vi "Parse IDN String.vi"(5 "error in (no error)":errorcluster, 6 "IDN String":string) -> (0 "error out":errorcluster, 1 "Info":string, 2 "Model":string, 3 "Manufacturer":string, 4 "Revision":string)   [LabVIEW 2019]
uses:
  New NML Data Acq/SubVIs/NML Data Acq Globals.vi
  <vilib>/regexp/Match Regular Expression.xnode
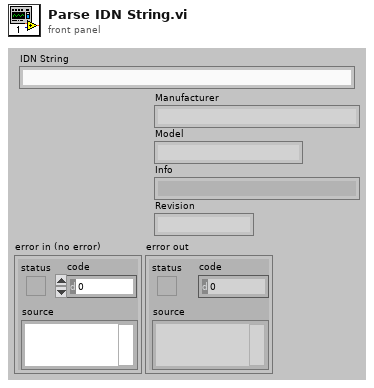
[diagram p1: front panel]
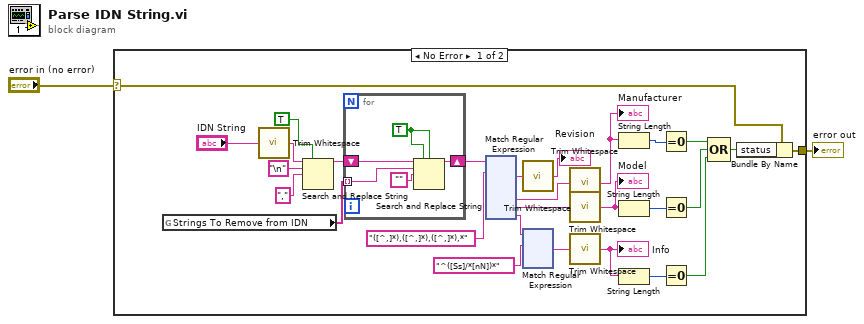
[diagram p0: block diagram]
diagram:
  n1 = case shown="No Error" "error in (no error)" {
    selector: "error in (no error)" -> [w24 w262]
    tunnel: [w23 w262] -> w1
    frame No Error {
      n2 = global read "NML Data Acq Globals.vi" "Strings To Remove from IDN"() -> (w22:string[])
      n3 = call <vilib>:"Trim Whitespace.vi"("string"="IDN String") -> ("trimmed string"=w3:string)  [unwired: 1 in]
      n4 = Search and Replace String(replace all?=TRUE ("replace all? (F)"), input string=w3, search string="\n", replace string="," ("replace string (\"\")")) -> (result string=w26:string)  [unwired: 4 in, 3 out]
      n5 = for {
        tunnel: w22 -> [w259] mode=indexing
        shift-right: [w260] -> w9
        shift-left: w26 -> [w261]
        w258 = TRUE ("replace all? (F)")
        n6 = Search and Replace String(replace all?=w258, case sensitive?=w258, input string=w261, search string=w259, replace string="") -> (result string=w260:string)  [unwired: 3 in, 3 out]
      }
      n7 = xnode "Match Regular Expression"("input string"=w9, "regular expression"="([^,]*),([^,]*),([^,]*),*" ("format string")) -> ("after match"=w10:string, "submatch 1"=w7:string, "submatch 2"=w6:string, "submatch 3"=w5:string)  [unwired: 4 in, 4 out]
      n8 = call <vilib>:"Trim Whitespace.vi"("string"=w10) -> ("trimmed string"=→"Revision":string)  [unwired: 1 in]
      n9 = xnode "Match Regular Expression"("input string"=w5, "regular expression"="^([Ss]/*[nN])*") -> ("after match"=w16:string)  [unwired: 4 in, 4 out]
      n10 = call <vilib>:"Trim Whitespace.vi"("string"=w7) -> ("trimmed string"=w20:string)  [unwired: 1 in]
      "Manufacturer" <- w20
      n11 = call <vilib>:"Trim Whitespace.vi"("string"=w6) -> ("trimmed string"=w15:string)  [unwired: 1 in]
      "Model" <- w15
      n12 = call <vilib>:"Trim Whitespace.vi"("string"=w16) -> ("trimmed string"=w4:string)  [unwired: 1 in]
      "Info" <- w4
      n13 = String Length(string=w20) -> (length=w21:i32)
      n14 = String Length(string=w15) -> (length=w19:i32)
      n15 = String Length(string=w4) -> (length=w18:i32)
      n16 = Equal To 0?(x=w21) -> (x = 0?=w12:bool)
      n17 = Equal To 0?(x=w19) -> (x = 0?=w13:bool)
      n18 = Equal To 0?(x=w18) -> (x = 0?=w11:bool)
      n19 = Compound Arithmetic op=OR(w12, w13, w11) -> (w14:bool)
      n20 = Bundle By Name(cluster=w24, "status"=w14) -> (w23:errorcluster)
    }
    frame Error {
    }
  }
  "error out" <- w1
